vi "dscADScanAvg.vi"(8 "error in":errorcluster, 9 "count":i32, 10 "dscadscan":T1, 11 "board":i16) -> (0 "error out":errorcluster, 2 "DataOut":cluster{"time":timestamp, "sample_val":sgl[]}, 3 "boardOut":i16)   [LabVIEW 2011, in "Diamond Universal Driver.lvlib"]
doc: "Performs AD conversion on each channel in the selected range. Channels are individually sampled in rapid sequence, not simultaneously. The samples are averaged and returned. \n\nFunction returns DE_OPERATION_TIMED_OOUT if a timeout occurs because the A/D circuit is not ready. This usually indicates a hardware error."
uses:
  Diamond Universal Driver.lvlib
  Controls/dscADScan.ctl
  Controls/gain.ctl
  Controls/error codes.ctl
  Instruments/WL OPC/Support/dlls/dscud.dll
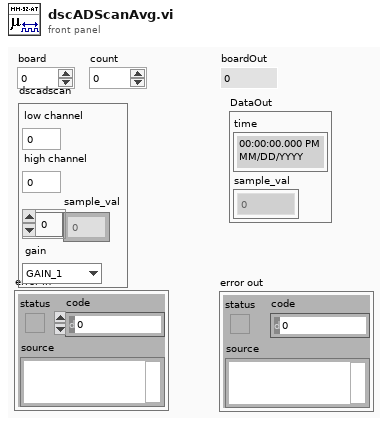
[diagram p1: front panel]
types:
  T1 = typedef "dscADScan.ctl" = cluster{"low channel":u8, "high channel":u8, "sample_val":u16[], "gain":T2}
  T2 = typedef "gain.ctl" = enum8{"GAIN_1", "GAIN_2", "GAIN_8"}
  T3 = typedef "Diamond Universal Driver.lvlib/error codes.ctl" = enum8{"DE_NONE", "DE_HW_FAILURE", "DE_SW_FAILURE", "DE_HW_NOT_SUPPORTED", "DE_SW_NOT_SUPPORTED", "DE_INVALID_PARM", "DE_ALTERNATE_IN_PROGRESS", "DE_NONE_IN_PROGRESS", "DE_BUFFER_ROLLOVER", "DE_INVALID_ERROR_CODE", "DE_ALREADY_PAUSED", "DE_OVERFLOW", "DE_INVALID_FUNC", "DE_DSCUDH_INVALID", "DE_INVALID_BOARD", "DE_BOARD_LIMIT_REACHED", "DE_BOARD_BUSY", "DE_INVALID_WINDRVR_HANDLE", "DE_INVALID_WINDRVR_VERSION", "DE_BAD_WINDRVR_BOARD_INIT", "DE_OPERATION_TIMED_OUT", "DE_INVALID_WINDRVR_KP", "DE_THREAD_FAILURE"}
  T4 = cluster{"seconds since 1Jan1904":timestamp, "sample_val":sgl[]}
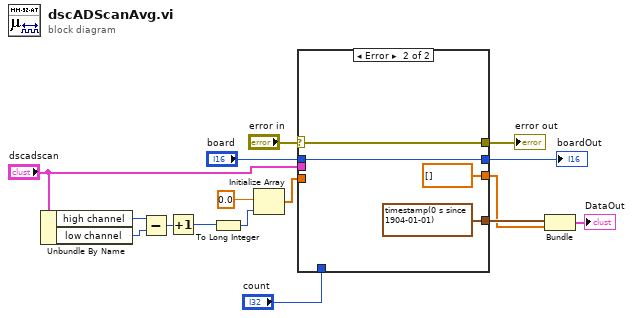
[diagram p0: block diagram]
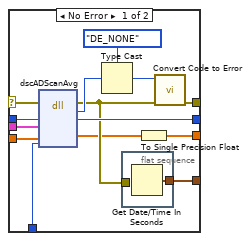
[diagram p2: hidden frame]
diagram:
  n1 = Unbundle By Name("dscadscan") -> ("high channel"=w10:u8, "low channel"=w9:u8)
  n2 = Subtract(x=w10, y=w9) -> (x-y=w7:u8)
  n3 = Increment(x=w7) -> (x+1=w6:u8)
  n4 = To Long Integer(number=w6) -> (32bit integer=w5:i32)
  n5 = Initialize Array(0.0, w5) -> (w11:dbl[])
  n6 = case shown="Error" "error in" {
    selector: "error in" -> [w30 w35]
    tunnel: [w26 w35] -> w15
    tunnel: [w25 w34] -> w14
    tunnel: "board" -> [w24 w34]
    tunnel: w11 -> [w21 _]
    tunnel: [w17 sgl[] [] ("sample_val")] -> w2
    tunnel: "dscadscan" -> [w23 _]
    tunnel: "count" -> [w22 _]
    tunnel: [w19 timestamp(0 s since 1904-01-01) ("seconds since 1Jan1904")] -> w3
    frame No Error {
      n7 = dll-call lib="C:/Users/mrichardson/Documents/Web Based Version Control SW/Instruments/WL OPC/Support/dlls/dscud.dll" fn="dscADScanAvg"(error in=w30, "board"=w24, "dscadscan"=w23, "sample_val"=w21, "count"=w22) -> (error out=w20:errorcluster, "error"=w29:u8, "board"=w25:i16, "sample_val"=w18:dbl[])  [unwired: 4 in, 1 out]
      n8 = Type Cast(type=error_codes."DE_NONE" ("error codes"), x=w29) -> (*(type *) &x=w27:T3)
      n9 = flat-sequence {
        tunnel: w20 -> [_]
        tunnel: [w31] -> w19
        frame #0 {
          n10 = Get Date/Time In Seconds() -> (seconds since 1Jan1904=w31:timestamp)
        }
      }
      n11 = To Single Precision Float(number=w18) -> (single precision float=w17:sgl[])
      n12 = call "Convert Code to Error.vi"("error in"=w20, "error codes"=w27) -> ("error out"=w26:errorcluster)  [unwired: 9 in]
    }
    frame Error {
    }
  }
  "error out" <- w15
  "boardOut" <- w14
  n13 = Bundle("seconds since 1Jan1904"=w3, "sample_val"=w2) -> (→"DataOut":T4)  [unwired: 1 in]
